vi "ParseDataMsg.vi"(8 "error in (no error)":errorcluster, 10 "JSON<>":string, 11 "Counter in":refnum<class "Counter.lvclass">) -> (0 "error out":errorcluster, 3 "Counter out":refnum<class "Counter.lvclass">)   [LabVIEW 2020, in "TestProcesses.lvlib" / "Counter.lvclass"]
uses:
  Counter.lvclass
  Counter.lvclass/Counter.ctl
  <vilib>/JDP Science/JSONtext/JSON text to Variant.vi
  a9a0de8f-4dcc-4ed7-ae3a-572a6b301798.vi
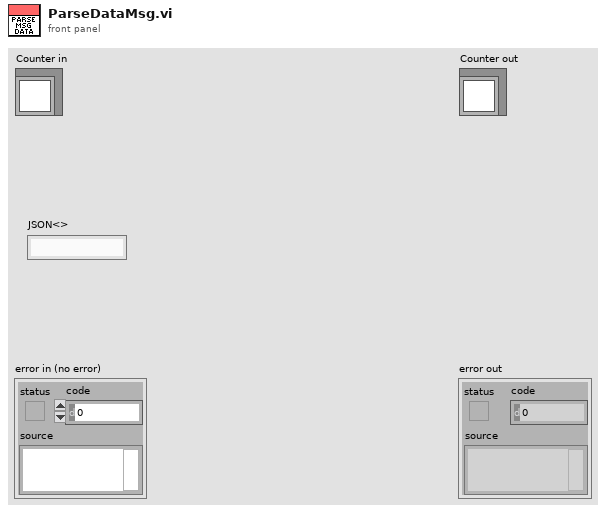
[diagram p1: front panel]
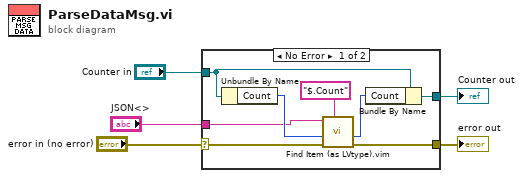
[diagram p0: block diagram]
diagram:
  n1 = case shown="No Error" "error in (no error)" {
    selector: "error in (no error)" -> [w9 w15]
    tunnel: [w8 w15] -> w5
    tunnel: [w13 w14] -> w4
    tunnel: "Counter in" -> [w12 w14]
    tunnel: "JSON<>" -> [w10 _]
    frame No Error {
      n2 = Unbundle By Name(w12) -> ("Count"=w11:u32)
      n3 = call "Find Item (as LVtype).vim"("$Path or Item Name"="$.Count", "error in (no error)"=w9, "Data Type and Default Value"=w11, "JSON"=w10) -> ("error out"=w8:errorcluster, "Data"=w6:u32)  [unwired: 4 in, 2 out]
      n4 = Bundle By Name(cluster=w12, "Count"=w6) -> (w13:refnum<class "Counter.lvclass">)
    }
    frame Error {
    }
  }
  "error out" <- w5
  "Counter out" <- w4
